vi "Get Status.vi"(8 "error in (no error)":errorcluster, 11 "CCD in":refnum<class "CCD.lvclass">) -> (0 "error out":errorcluster, 2 "Camera Status":T1, 3 "CCD out":refnum<class "CCD.lvclass">)   [LabVIEW 2018, in "CCD.lvclass"]
uses:
  CCD.lvclass
  CCD.lvclass/CCD.ctl
  Cooler/Cooler.lvclass
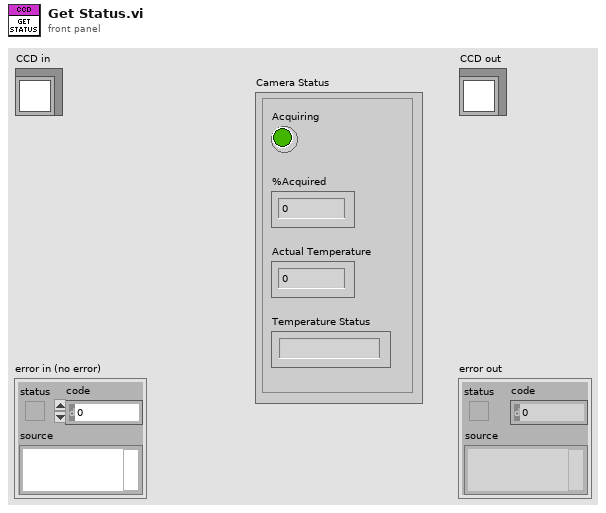
[diagram p1: front panel]
types:
  T1 = cluster{"Acquiring":bool, "%Acquired":dbl, "Actual Temperature":i16, "Temperature Status":string}
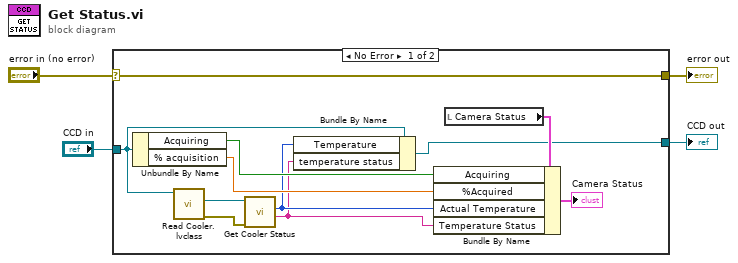
[diagram p0: block diagram]
diagram:
  n1 = case shown="No Error" "error in (no error)" {
    selector: "error in (no error)" -> [w15 w17]
    tunnel: [w15 w17] -> w3
    tunnel: [w7 w16] -> w1
    tunnel: "CCD in" -> [w8 w16]
    frame No Error {
      n2 = Unbundle By Name(w8) -> ("Acquiring"=w10:bool, "% acquisition"=w9:dbl)
      n3 = call "Read Cooler.lvclass.vi"("CCD in"=w8) -> ("error out"=w13:errorcluster, "Cooler.lvclass"=w14:refnum<class "Cooler.lvclass">)  [unwired: 8 in, 1 out]
      n4 = call "Get Cooler Status.vi"("error in (no error)"=w13, "Cooler in"=w14) -> ("Temperature Status"=w5:string, "Temperature"=w6:i16)  [unwired: 6 in, 2 out]
      n5 = Bundle By Name(cluster=w8, "Temperature"=w6, "temperature status"=w5) -> (w7:refnum<class "CCD.lvclass">)
      n6 = local read "Camera Status"() -> (w11:T1)
      n7 = Bundle By Name(cluster=w11, "Acquiring"=w10, "%Acquired"=w9, "Actual Temperature"=w6, "Temperature Status"=w5) -> (→"Camera Status":T1)
    }
    frame Error {
    }
  }
  "error out" <- w3
  "CCD out" <- w1
